vi "WebSockets Server.vi"() -> ()   [LabVIEW 2020]
uses:
  Type Defs/State.ctl
  <vilib>/MediaMongrels Ltd/WebSockets/WebSockets/WebSocket Server/WebSocket Server.lvclass
  <vilib>/MediaMongrels Ltd/WebSockets/Sockets/VISA TCP Listener/VISA TCP Listener.lvclass
  <vilib>/MakerHub/LINX/Public/Utilities/Open Local.vi
  <vilib>/MakerHub/LINX/LMH-LINX.lvlib
panel:
  out "Data":string
  out "Device IP Address":string
  in  "Stop":bool
  out "Current Time":string
  # "TCP Port 6123"
  # "ws://host:port"
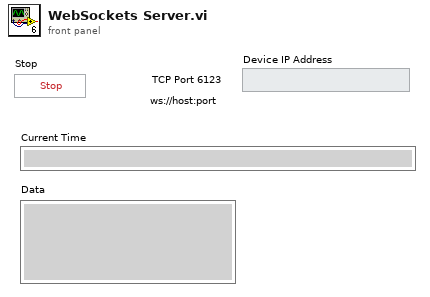
[diagram p1: front panel]
types:
  T1 = typedef "State.ctl" = enum16{"Initialise", "Listen", "Write Data", "Read Data", "Running", "Close WebSocket", "Exit"}
  T2 = typedef "LMH-LINX.lvlib/LINX Ref.ctl" = cluster{"IO":T3, "Interface":T4, "LINX Device Config":T5}
  T3 = typedef "LMH-LINX.lvlib/Platform.ctl" = enum16{"Remote", "Local"}
  T4 = typedef "LMH-LINX.lvlib/Interface.ctl" = enum16{"Serial", "TCP"}
  T5 = typedef "LMH-LINX.lvlib/Device.lvlib/LINX Device Config.ctl" = cluster{"Interface":T4, "COM Port":refnum<visa-resource-name>, "TCP Configuration":T6, "Device Family":u8, "Device ID":u8, "Device Name":string, "TCP Ref":refnum<k5>, "Channels":T7}
  T6 = typedef "LMH-LINX.lvlib/Device.lvlib/TCP Config.ctl" = cluster{"IP Address":string, "Port":u16}
  T7 = typedef "LMH-LINX.lvlib/Channels.ctl" = cluster{"DI":u8[], "DO":u8[], "AI":u8[], "AO":u8[], "PWM":u8[], "QE":u8[], "UART":u8[], "I2C 2":u8[], "SPI":u8[], "CAN":u8[], "Servo":u8[], "AI Ref (V)":dbl, "AI Resolution (Bits)":u8, "AO Ref (V)":dbl, "AO Resolution (Bits)":u8}
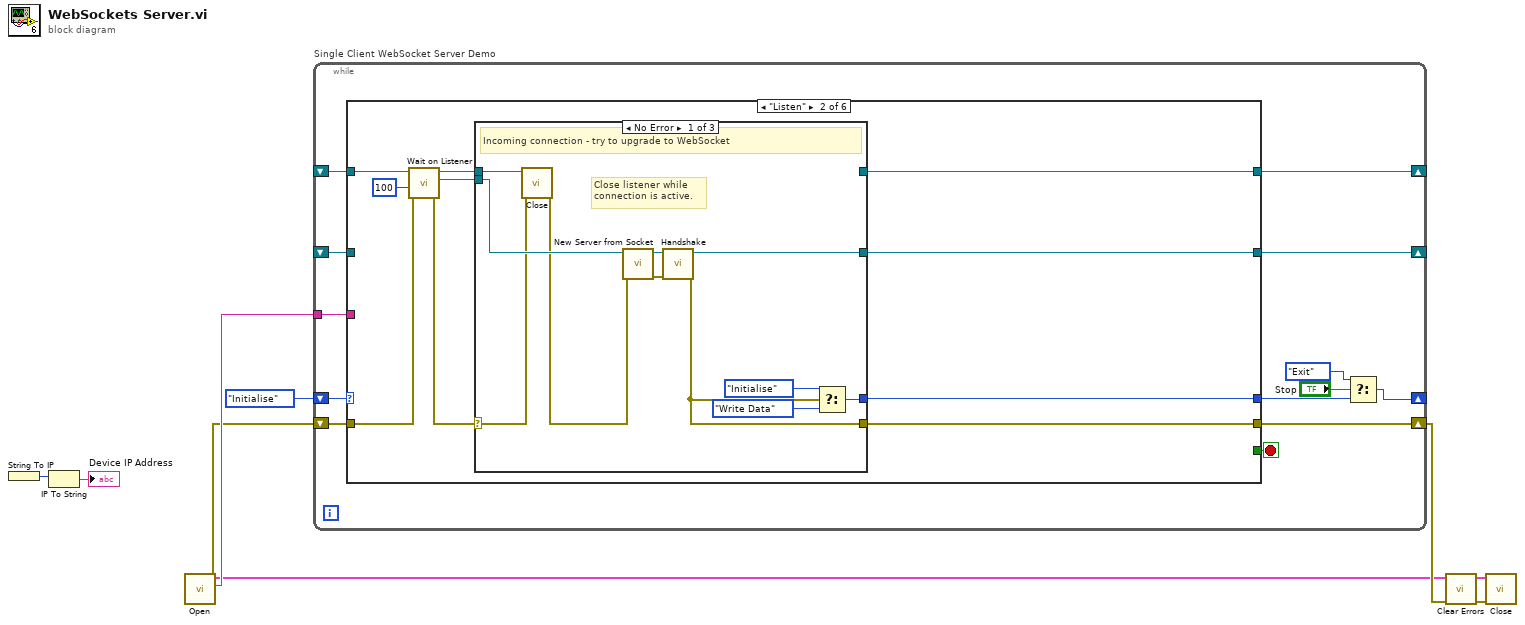
[diagram p0: block diagram]
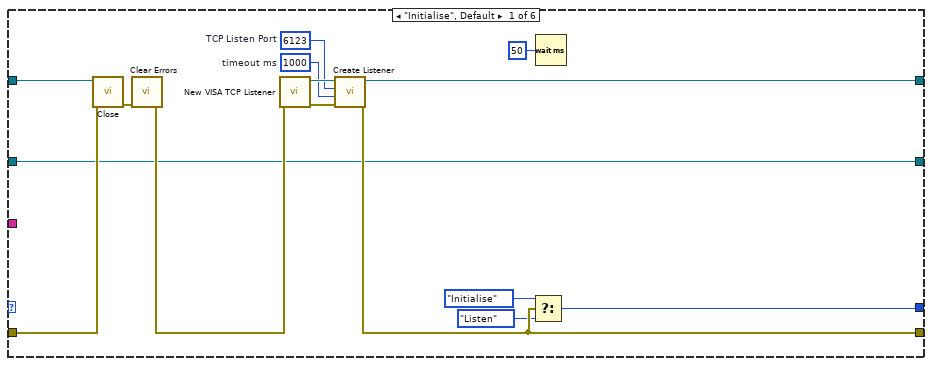
[diagram p2: hidden frame]
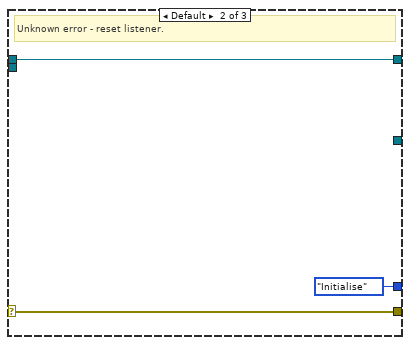
[diagram p3: hidden frame]
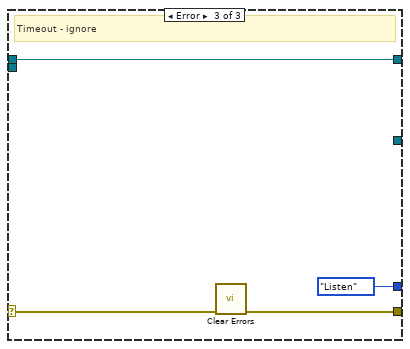
[diagram p4: hidden frame]
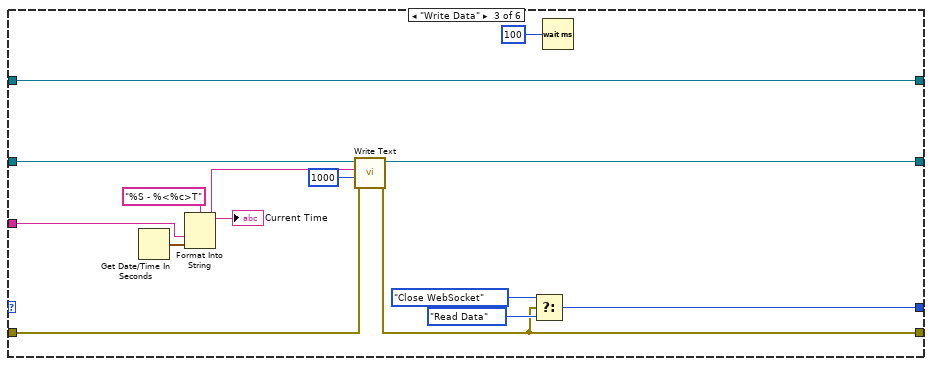
[diagram p5: hidden frame]
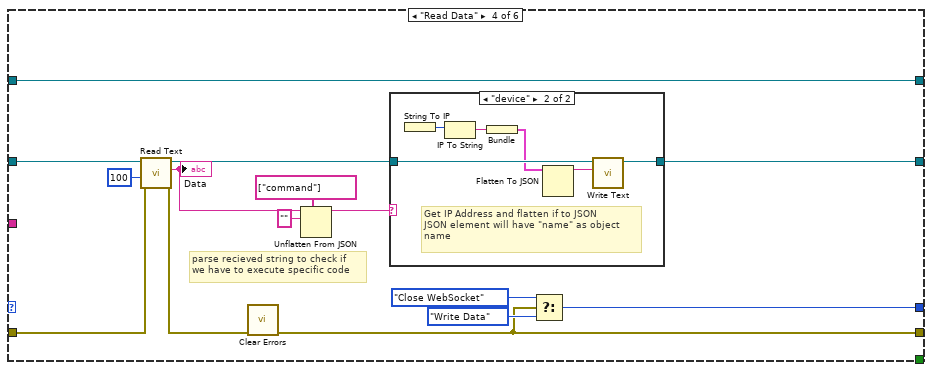
[diagram p6: hidden frame]
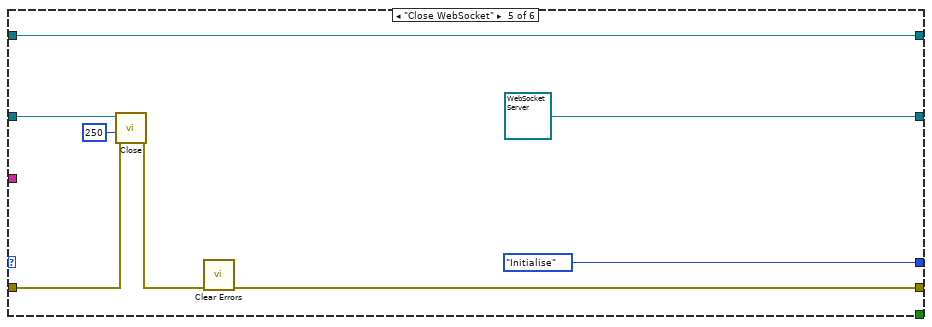
[diagram p8: hidden frame]
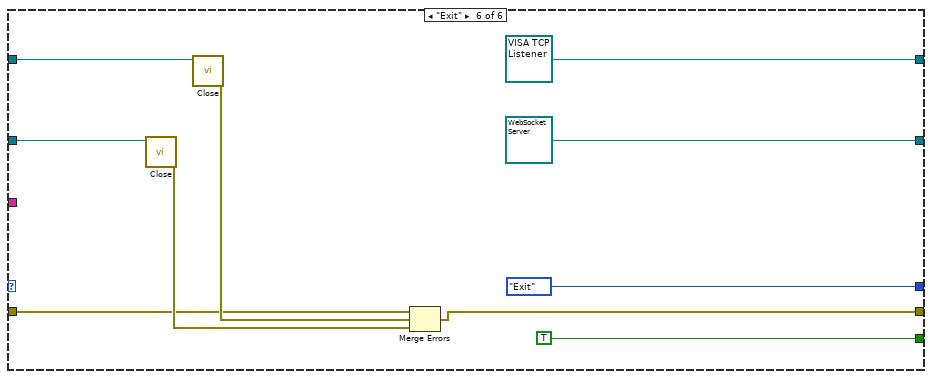
[diagram p9: hidden frame]
diagram:
  n1 = String To IP() -> (0:w7:u32)  [unwired: 1 in]
  n2 = IP To String(2:w7) -> (0:→"Device IP Address":string)  [unwired: 1 in]
  n3 = call-poly <vilib>:"Open.vi"() -> ("Error Out"=w4:errorcluster, "Device Name"=w5:string, "LINX Resource"=w2:T2)  [unwired: 9 in]
  n4 = while "Single Client WebSocket Server Demo" {
    shift-right: [w10] -> _
    shift-left: State."Initialise" ("Enum") -> [w21]
    shift-right: [w19] -> _
    shift-left: _ -> [w14]
    shift-right: [w18] -> w3
    shift-left: w4 -> [w17]
    shift-right: [w16] -> _
    shift-left: _ -> [w15]
    tunnel: w5 -> [w9]
    stop <- w20 stop-if-true
    n5 = case shown="\"Listen\"" w21 {
      tunnel: [_ _ _ _ _ TRUE] -> w20
      tunnel: [w26 w38 w77 w92 State."Initialise" ("Enum") State."Exit" ("Enum")] -> w11
      tunnel: [w30 w41 w78 w93 w101 refnum<class "VISA TCP Listener.lvclass"> refnum ("VISA TCP Listener out")] -> w19
      tunnel: w14 -> [w29 w42 w78 w93 w101 w114]
      tunnel: [w27 w39 w68 w85 w104 w111] -> w18
      tunnel: w17 -> [w28 w40 w69 w88 w105 w112]
      tunnel: [w22 w37 w65 w79 refnum<class "WebSocket Server.lvclass"> refnum ("WebSocket out") refnum<class "WebSocket Server.lvclass"> refnum ("WebSocket out")] -> w16
      tunnel: w15 -> [w22 _ w70 w89 w106 w113]
      tunnel: w9 -> [_ _ w66 _ _ _]
      frame "Initialise", Default {
        w33 = 1000  # timeout ms
        w34 = u16 6123  # TCP Listen Port
        n6 = call-dynamic <vilib>:"Close.vi"("error in (no error)"=w28, "VISA TCP Listener in"=w29) -> ("error out"=w32:errorcluster)  [unwired: 9 in]
        n7 = call <vilib>:"Clear Errors.vi"("error in (no error)"=w32) -> ("error out"=w31:errorcluster)  [unwired: 5 in, 1 out]
        n8 = call <vilib>:"New VISA TCP Listener.vi"("error in (no error)"=w31) -> ("error out"=w35:errorcluster, "VISA TCP Listener out"=w36:refnum<class "VISA TCP Listener.lvclass">)  [unwired: 9 in]
        n9 = call-dynamic "Create Listener.vi"("error in (no error)"=w35, "timeout ms (5000)"=w33, "Port"=w34, "VISA TCP Listener in"=w36) -> ("error out"=w27:errorcluster, "VISA TCP Listener out"=w30:refnum<class "VISA TCP Listener.lvclass">)  [unwired: 6 in]
        n10 = Select(t=State."Initialise" ("Enum"), s=w27, f=State."Listen" ("Enum")) -> (s? t:f=w26:T1)
        n11 = Wait (ms)(milliseconds to wait=u32 50) -> ()  [unwired: 1 out]
      }
      frame "Listen" {
        n12 = call-dynamic "Wait on Listener.vi"("error in (no error)"=w40, "timeout ms (5000)"=100, "VISA TCP Listener in"=w42) -> ("error out"=w45:errorcluster, "Socket out"=w46:refnum<class "Socket.lvclass">, "VISA TCP Listener out"=w44:refnum<class "VISA TCP Listener.lvclass">)  [unwired: 6 in]
        n13 = case shown="No Error" w45 {
          selector: w45 -> [w53 w60 w64]
          tunnel: w46 -> [w55 _ _]
          tunnel: w44 -> [w52 w59 w63]
          tunnel: [w51 _ _] -> w37
          tunnel: [w50 w60 w61] -> w39
          tunnel: [_ w59 w63] -> w41
          tunnel: [w48 State."Initialise" State."Listen"] -> w38
          frame No Error {
            # "Close listener while connection is active."
            # "Incoming connection - try to upgrade to WebSocket"
            n14 = call-dynamic <vilib>:"Close.vi"("error in (no error)"=w53, "VISA TCP Listener in"=w52) -> ("error out"=w54:errorcluster)  [unwired: 9 in]
            n15 = call <vilib>:"New Server from Socket.vi"("error in (no error)"=w54, "Socket"=w55) -> ("error out"=w56:errorcluster, "WebSocket Server out"=w57:refnum<class "WebSocket Server.lvclass">)  [unwired: 8 in]
            n16 = call-dynamic "Handshake.vi"("error in (no error)"=w56, "WebSocket Connection in"=w57) -> ("error out"=w50:errorcluster, "WebSocket Connection out"=w51:refnum<class "WebSocket Server.lvclass">)  [unwired: 8 in]
            n17 = Select(t=State."Initialise", s=w50, f=State."Write Data") -> (s? t:f=w48:T1)
          }
          frame Default {
            # "Unknown error - reset listener."
          }
          frame Error {
            # "Timeout - ignore"
            n18 = call <vilib>:"Clear Errors.vi"("error in (no error)"=w64) -> ("error out"=w61:errorcluster)  [unwired: 5 in, 1 out]
          }
        }
      }
      frame "Write Data" {
        n19 = Get Date/Time In Seconds() -> (seconds since 1Jan1904=w67:timestamp)
        n20 = Format Into String(format string="%S - %<%c>T", w66, w67) -> (resulting string=w73:string)  [unwired: 2 in, 1 out]
        "Current Time" <- w73
        n21 = call-dynamic "Write Text.vi"("error in (no error)"=w69, "timeout ms (5000)"=1000, "String Data"=w73, "WebSocket in"=w70) -> ("error out"=w68:errorcluster, "WebSocket out"=w65:refnum<class "WebSocket Server.lvclass">)  [unwired: 6 in]
        n22 = Select(t=State."Close WebSocket" ("Enum"), s=w68, f=State."Read Data" ("Enum")) -> (s? t:f=w77:T1)
        n23 = Wait (ms)(milliseconds to wait=u32 100) -> ()  [unwired: 1 out]
      }
      frame "Read Data" {
        # "parse recieved string to check if \nwe have to execute specific code"
        n24 = call-dynamic "Read Text.vi"("error in (no error)"=w88, "timeout ms (5000)"=100, "WebSocket in"=w89) -> ("error out"=w87:errorcluster, "Data"=w84:string, "WebSocket out"=w80:refnum<class "WebSocket Server.lvclass">)  [unwired: 6 in]
        "Data" <- w84
        n25 = call <vilib>:"Clear Errors.vi"("error in (no error)"=w87) -> ("error out"=w85:errorcluster)  [unwired: 5 in, 1 out]
        n26 = Unflatten From JSON(path=string[] ["command"], JSON string=w84, type and defaults="") -> (value=w83:string)  [unwired: 4 in, 1 out]
        n27 = case shown="\"device\"" w83 {
          tunnel: w80 -> [w94 w99]
          tunnel: [w94 w98] -> w79
          frame "False", Default {
          }
          frame "device" {
            # "Get IP Address and flatten if to JSON\nJSON element will have \"name\" as object\nname"
            n28 = String To IP() -> (0:w100:u32)  [unwired: 1 in]
            n29 = IP To String(2:w100) -> (0:w97:string)  [unwired: 1 in]
            n30 = Bundle("name"=w97) -> (w96:cluster{"name":string})  [unwired: 1 in]
            n31 = Flatten To JSON(anything=w96) -> (JSON string=w95:string)  [unwired: 2 in, 1 out]
            n32 = call-dynamic "Write Text.vi"("String Data"=w95, "WebSocket in"=w99) -> ("WebSocket out"=w98:refnum<class "WebSocket Server.lvclass">)  [unwired: 8 in, 1 out]
          }
        }
        n33 = Select(t=State."Close WebSocket" ("Enum"), s=w85, f=State."Write Data" ("Enum")) -> (s? t:f=w92:T1)
      }
      frame "Close WebSocket" {
        n34 = call-dynamic <vilib>:"Close.vi"("error in (no error)"=w105, "timeout ms (5000)"=250, "WebSocket in"=w106) -> ("error out"=w107:errorcluster)  [unwired: 8 in]
        n35 = call <vilib>:"Clear Errors.vi"("error in (no error)"=w107) -> ("error out"=w104:errorcluster)  [unwired: 5 in, 1 out]
      }
      frame "Exit" {
        n36 = call-dynamic <vilib>:"Close.vi"("WebSocket in"=w113) -> ("error out"=w116:errorcluster)  [unwired: 10 in]
        n37 = call-dynamic <vilib>:"Close.vi"("VISA TCP Listener in"=w114) -> ("error out"=w115:errorcluster)  [unwired: 10 in]
        n38 = Merge Errors(w112, w115, w116) -> (w111:errorcluster)
      }
    }
    n39 = Select(t=State."Exit" ("Enum"), s="Stop", f=w11) -> (s? t:f=w10:T1)
  }
  n40 = call <vilib>:"Clear Errors.vi"("error in (no error)"=w3) -> ("error out"=w1:errorcluster)  [unwired: 5 in, 1 out]
  n41 = call <vilib>:"Close.vi"("Error In"=w1, "LINX Resource"=w2) -> ()  [unwired: 9 in, 1 out]
